vi "Non Callback Test.vi"() -> ()   [LabVIEW 2011]
uses:
  DepthSense State.ctl
  <vilib>/Platform/TimedLoop/XDataNode/timing_clust.ctl
  <vilib>/Platform/TimedLoop/XDataNode/nitl_modes.ctl
  <vilib>/Platform/TimedLoop/XDataNode/wakeup.ctl
  <vilib>/vision/Image Controls.llb/IMAQ Image.ctl
  C:/Users/Behavior Room/Desktop/Kinect Mouse/DepthSense/FunctionPointerProxy/FunctionPointerProxy/bin/Release/FunctionPointerProxy.dll
  FunctionPointerProxy/FunctionPointerProxy/bin/Release/FunctionPointerProxy.dll
  DepthSense Global Status.vi
  <vilib>/Platform/TimedLoop/XDataNode/XDataNode.xnode
  <userlib>/libOptrima-2-3/libOptrima-2-3.lvlib
  Program Files (x86)/SoftKinetic/OptrimaSDK/lib/libOptrima-2-3.dll
  <vilib>/Platform/TimedLoop/XDataNode/XDNodeRunTimeDep.lvlib
panel:
  out "NewFrame Callback?":i32
  out "Image":T1(plugin-control)
  in  "DepthSense Local Status":T2={"Camera Version"="", "Image Height"=0, "Image Width"=0, "Minimum Framerate"=0, "Maximum Framerate"=0, "Framerate"=25, "Close Mode"=FALSE, "Denoising"=TRUE, "Leakage Algorithm"=TRUE, "Anti-Aliasing"=TRUE, "Camera Status"=-2, "API Version"="", "Light Intensity"=100}
  in  "stop":bool
  out "Connect Callback?":i32
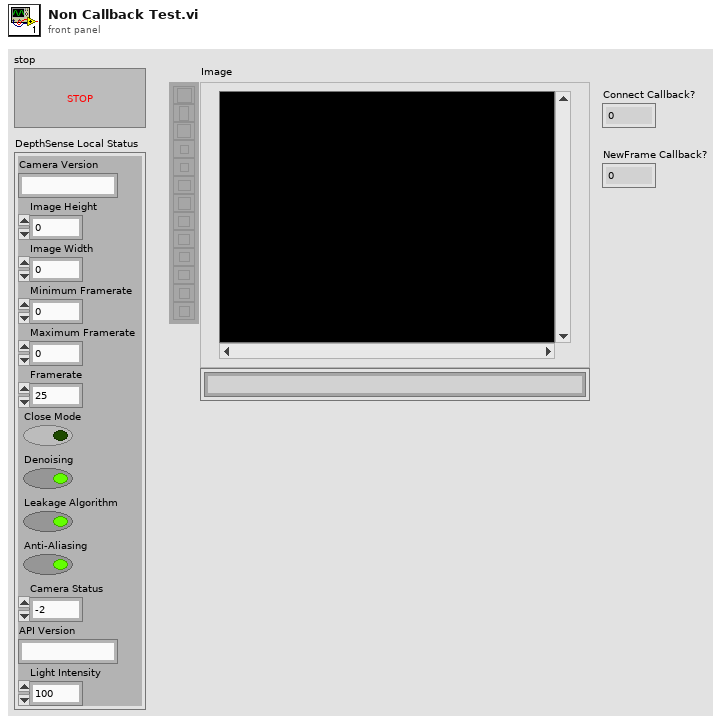
[diagram p1: front panel]
types:
  T1 = typedef "IMAQ Image.ctl" = refnum<image>
  T2 = typedef "DepthSense State.ctl" = cluster{"Camera Version":string, "Image Height":i32, "Image Width":i32, "Minimum Framerate":i32, "Maximum Framerate":i32, "Framerate":i32, "Close Mode":bool, "Denoising":bool, "Leakage Algorithm":bool, "Anti-Aliasing":bool, "Camera Status":i32, "API Version":string, "Light Intensity":i32}
  T3 = typedef "t_CallbackReferences.ctl" = cluster{"LV event callback ":refnum<k27>, "Proxy instance":refnum<k24>, "(*f)(...)":i32}
  T4 = typedef "XDNodeRunTimeDep.lvlib/timing_clust.ctl" = cluster{"Expected End [f-1]":u64, "Actual End [f-1]":u64, "Finished Late? [f-1]":bool, "Expected End [i-1]":u64, "Actual End [i-1]":u64, "Finished Late? [i-1]":bool, "Expected Start [i]":u64, "Actual Start [i]":u64, "Expected Start [f]":u64, "Actual Start [f]":u64, "Source Name":string, "Structure Name":string, "Period":i64, "Deadline":i64, "Offset":i64, "Start":i64, "Priority":i32, "Timeout":i32, "Mode":T5, "Wakeup Reason":T6, "Error":errorcluster, "Source Type":string, "Secondary Source Type":string, "Global End Time":u64, "Global Start Time":u64, "Frame Duration":u64, "Iteration Duration":u64, "Assigned CPU":i32, "I/O Scan Engine Mode":u32}
  T5 = typedef "XDNodeRunTimeDep.lvlib/nitl_modes.ctl" = enum32{"No Change", "Process missed periods, maintain original phase", "Discard missed periods, maintain original phase", "Process missed periods, ignore original phase", "Discard missed periods, ignore original phase"}
  T6 = typedef "XDNodeRunTimeDep.lvlib/wakeup.ctl" = enum32{"Normal", "Aborted", "Asynchronous wakeup", "Timing source error", "Timed loop error", "Timeout"}
  T7 = typedef "Image Type" = u32
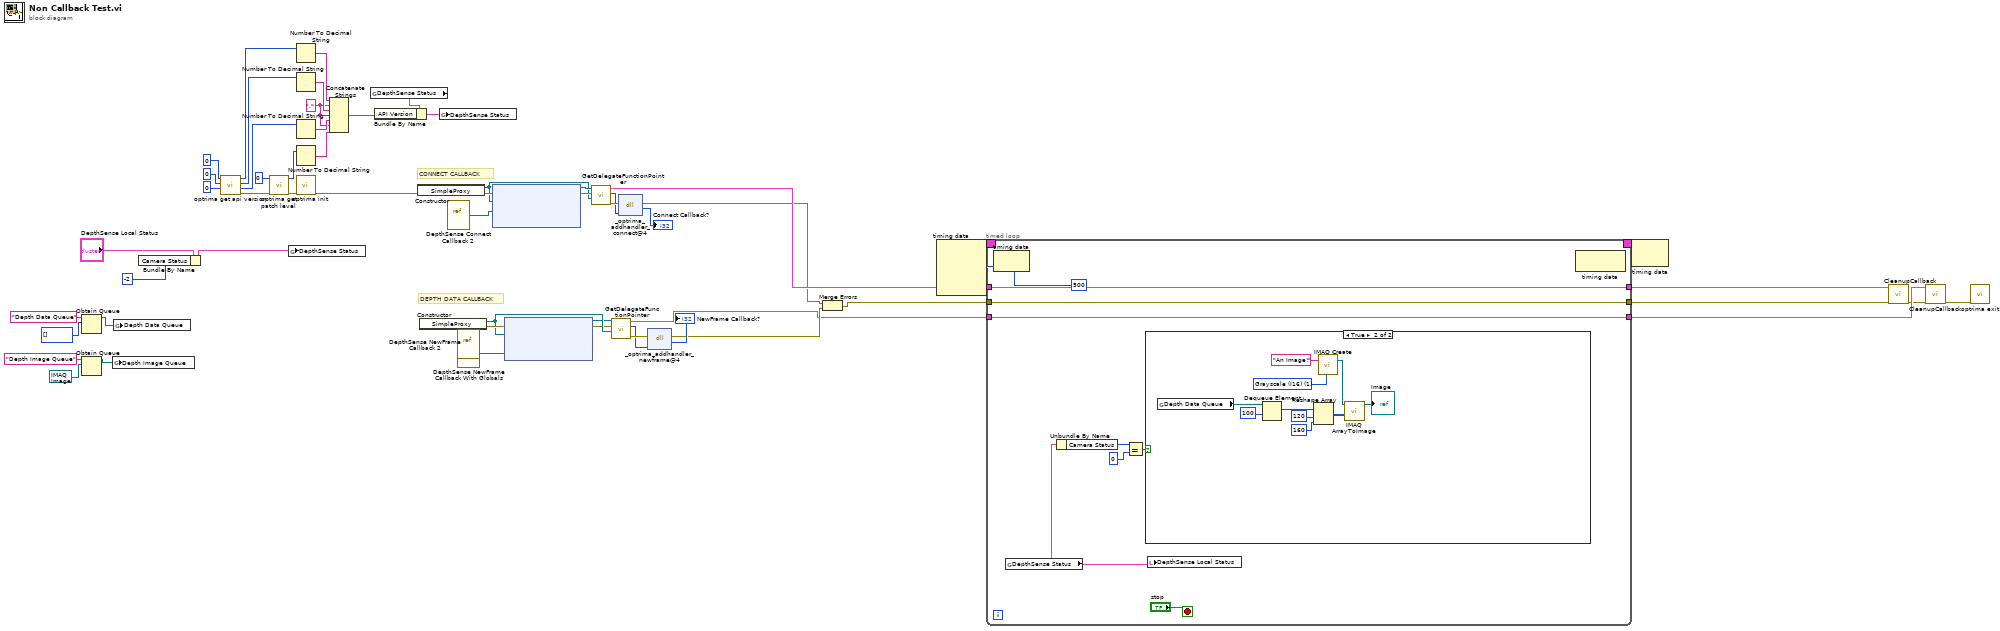
[diagram p0: block diagram]
diagram:
  w43 = "."
  # "DEPTH DATA CALLBACK"
  # "CONNECT CALLBACK"
  n1 = Obtain Queue(name (unnamed)="Depth Data Queue", element data type=u16[] [] ("p_depthmap in")) -> (queue out=w20:refnum<queue>)  [unwired: 3 in, 2 out]
  n2 = Obtain Queue(name (unnamed)="Depth Image Queue", element data type=T1 refnum ("New Image")) -> (queue out=w19:refnum<queue>)  [unwired: 3 in, 2 out]
  n3 = global write "DepthSense Global Status.vi" "Depth Image Queue"(w19) -> ()
  n4 = global write "DepthSense Global Status.vi" "Depth Data Queue"(w20) -> ()
  n5 = Bundle By Name(cluster="DepthSense Local Status", "Camera Status"=-2) -> (w29:T2)
  n6 = call <userlib>:"optrima get api version.vi"("minor"=u32 0, "major"=u32 0, "release"=u32 0) -> ("error out"=w57:errorcluster, "minor out"=w53:u32, "major out"=w54:u32, "release out"=w55:u32)  [unwired: 5 in]
  n7 = call <userlib>:"optrima get patch level.vi"("error in (no error)"=w57, "patch"=u32 0) -> ("error out"=w56:errorcluster, "patch out"=w52:u32)  [unwired: 8 in]
  n8 = global write "DepthSense Global Status.vi" "DepthSense Status"(w29) -> ()
  n9 = Number To Decimal String(number=w55) -> (decimal integer string=w51:string)  [unwired: 1 in]
  n10 = Number To Decimal String(number=w54) -> (decimal integer string=w46:string)  [unwired: 1 in]
  n11 = Number To Decimal String(number=w53) -> (decimal integer string=w45:string)  [unwired: 1 in]
  n12 = Number To Decimal String(number=w52) -> (decimal integer string=w44:string)  [unwired: 1 in]
  n13 = call <userlib>:"optrima init.vi"("error in (no error)"=w56) -> ("error out"=w35:errorcluster)  [unwired: 10 in]
  n14 = Concatenate Strings(w51, w43, w46, w43, w45, w43, w44) -> (w30:string)
  n15 = global read "DepthSense Global Status.vi" "DepthSense Status"() -> (w31:T2)
  n16 = Bundle By Name(cluster=w31, "API Version"=w30) -> (w32:T2)
  n17 = constructor class="SimpleProxy"(error in=w35) -> (reference out=w39:refnum<k24>, error out=w42:errorcluster)  [unwired: 2 in, 1 out]
  n18 = constructor class="SimpleProxy"() -> (reference out=w14:refnum<k24>, error out=w16:errorcluster)  [unwired: 3 in, 1 out]
  n19 = global write "DepthSense Global Status.vi" "DepthSense Status"(w32) -> ()
  n20 = vi-ref "DepthSense Connect Callback 2.vi"() -> ("vi reference"=w17:refnum<vi>)
  n21 = vi-ref "DepthSense NewFrame Callback 2.vi"() -> ()  [unwired: 1 out]
  n22 = vi-ref "DepthSense NewFrame Callback With Globals.vi"() -> ("vi reference"=w9:refnum<vi>)
  n23 = node(w42, w39, w17) -> (w41:refnum<k27>, w40:errorcluster)  [unwired: 2 in]
  n24 = node(w16, w14, w9) -> (w12:refnum<k27>, w13:errorcluster)  [unwired: 2 in]
  n25 = call "GetDelegateFunctionPointer.vi"("target class"=w39, "error in (no error)"=w40, "event callback refnum"=w41) -> ("error out"=w38:errorcluster, "(*f)(...)"=w37:i32, "References"=w34:T3)  [unwired: 6 in]
  n26 = call "GetDelegateFunctionPointer.vi"("target class"=w14, "error in (no error)"=w13, "event callback refnum"=w12) -> ("error out"=w11:errorcluster, "(*f)(...)"=w10:i32, "References"=w5:T3)  [unwired: 6 in]
  n27 = dll-call lib="C:/Program Files (x86)/SoftKinetic/OptrimaSDK/lib/libOptrima-2-3.dll" fn="_optrima_addhandler_connect@4"(error in=w38, "handlerfunc"=w37) -> (error out=w8:errorcluster, "return type"=→"Connect Callback?":i32)  [unwired: 3 in, 1 out]
  n28 = dll-call lib="C:/Program Files (x86)/SoftKinetic/OptrimaSDK/lib/libOptrima-2-3.dll" fn="_optrima_addhandler_newframe@4"(error in=w11, "handlerfunc"=w10) -> (error out=w7:errorcluster, "return type"=→"NewFrame Callback?":i32)  [unwired: 3 in, 1 out]
  n29 = Merge Errors(w8, w7) -> (w6:errorcluster)
  n30 = node-c288(i64 500 ("Period")) -> (w27:T4)  [unwired: 3 in]
  n31 = timed-loop {
    tunnel: [w65] -> w3
    tunnel: w6 -> [w65]
    tunnel: [w64] -> w18
    tunnel: w34 -> [w64]
    timing: w27 -> [_]
    timing-out: [_] -> w26
    tunnel: w5 -> [w58]
    tunnel: [w58] -> w4
    stop <- "stop" stop-if-true
    n32 = node-c288() -> ()  [unwired: 1 in, 1 out]
    n33 = global read "DepthSense Global Status.vi" "DepthSense Status"() -> (w62:T2)
    n34 = Unbundle By Name(w62) -> ("Camera Status"=w60:i32)
    n35 = Equal?(x=w60, y=0) -> (x = y?=w61:bool)
    n36 = case shown="True" w61 {
      frame False {
      }
      frame True {
        w76 = T7 1 items=["Grayscale (U8)", "Grayscale (I16)", "Grayscale (SGL)", "Complex (CSG)", "RGB (U32)", "HSL (U32)", "RGB (U64)", "Grayscale (U16)"] ("Image Type")
        n37 = global read "DepthSense Global Status.vi" "Depth Data Queue"() -> (w70:refnum<queue>)
        n38 = Dequeue Element(queue=w70, timeout in ms (-1)=100) -> (element=w68:u16[])  [unwired: 1 in, 3 out]
        n39 = Reshape Array(w68, 120 ("dimension size"), 160 ("dimension size")) -> (w72:u16[][])
        n40 = call "IMAQ Create"("Image Name"="An Image!", "Image Type"=w76) -> ("New Image"=w77:T1)  [unwired: 3 in, 1 out]
        n41 = call "IMAQ ArrayToImage"("Image Pixels (I16)"=w72, "Image"=w77) -> ("Image Out"=→"Image":T1)  [unwired: 8 in, 1 out]
      }
    }
    n42 = local write "DepthSense Local Status"(w62) -> ()
    n43 = node-c288() -> ()  [unwired: 1 in, 1 out]
  }
  n44 = node-c288(w26) -> ()  [unwired: 1 out]
  n45 = call "CleanupCallback.vi"("error in (no error)"=w3, "References"=w18) -> ("error out"=w2:errorcluster)  [unwired: 9 in]
  n46 = call "CleanupCallback.vi"("error in (no error)"=w2, "References"=w4) -> ("error out"=w1:errorcluster)  [unwired: 9 in]
  n47 = call <userlib>:"optrima exit.vi"("error in (no error)"=w1) -> ()  [unwired: 10 in, 1 out]
